vi "Calc Starting Conditions.vi"(9 "Reciprocals":T3, 10 "Middle":T1, 11 "Bottom":T1) -> (3 "Start Row Columns":T2, 5 "Start Row":i32)   [LabVIEW 2022 SP3, in "Raster.lvlib"]
uses:
  Raster.lvlib
  Point 2D.ctl
  Reciprocals.ctl
  Current Row.ctl
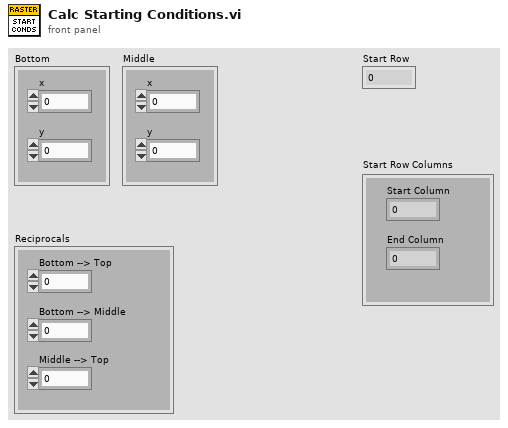
[diagram p1: front panel]
types:
  T1 = typedef "Raster.lvlib/Point 2D.ctl" = cluster{"x":i32, "y":i32}
  T2 = typedef "Raster.lvlib/Current Row.ctl" = cluster{"Start Column":sgl, "End Column":sgl}
  T3 = typedef "Raster.lvlib/Reciprocals.ctl" = cluster{"Bottom --> Top":sgl, "Bottom --> Middle":sgl, "Middle --> Top":sgl}
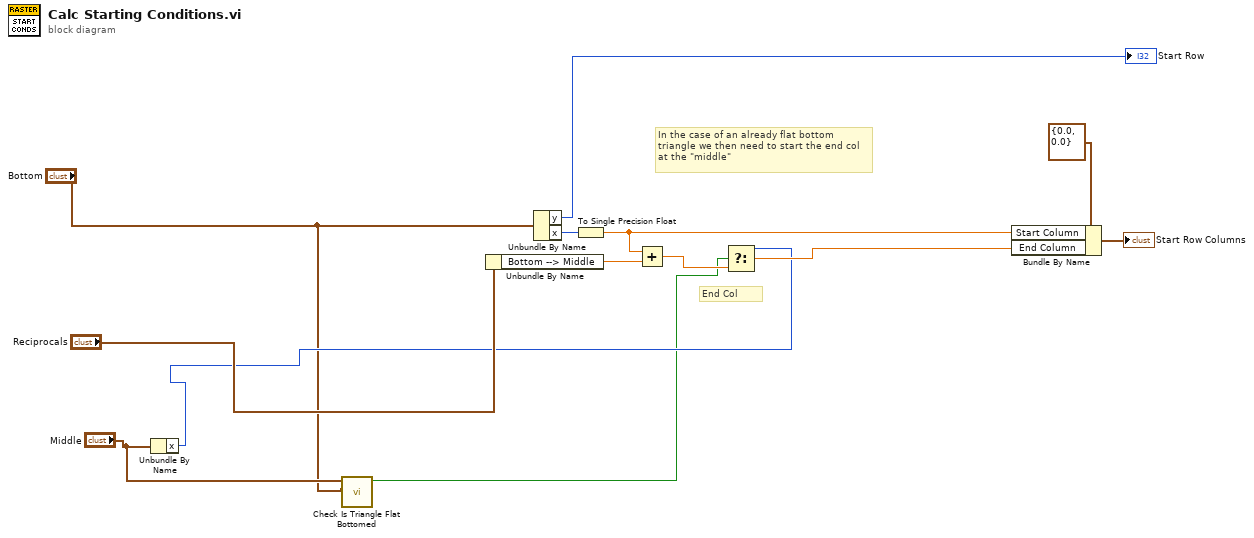
[diagram p0: block diagram]
diagram:
  # "End Col"
  # "In the case of an already flat bottom triangle we then need to start the end col at the \"middle\""
  n1 = Unbundle By Name("Middle") -> ("x"=w4:i32)
  n2 = call "Check Is Triangle Flat Bottomed.vi"("Bottom"="Bottom", "Middle"="Middle") -> ("Flat Bottom Triangle"=w1:bool)  [unwired: 9 in]
  n3 = Unbundle By Name("Reciprocals") -> ("Bottom --> Middle"=w13:sgl)
  n4 = Unbundle By Name("Bottom") -> ("y"=→"Start Row":i32, "x"=w10:i32)
  n5 = To Single Precision Float(number=w10) -> (single precision float=w6:sgl)
  n6 = Add(x=w6, y=w13) -> (x+y=w11:sgl)
  n7 = Select(t=w4, s=w1, f=w11) -> (s? t:f=w5:sgl)
  n8 = Bundle By Name(cluster=T2 {"Start Column"=0.0, "End Column"=0.0} ("Current Row"), "Start Column"=w6, "End Column"=w5) -> (→"Start Row Columns":T2)
